vi "DeMux4x4.vi"(1 "Data":bool[](array[boolean]), 2 "Select":bool[](array[boolean])) -> (0 "A":bool[][](array[boolean]))   [LabVIEW 2012]
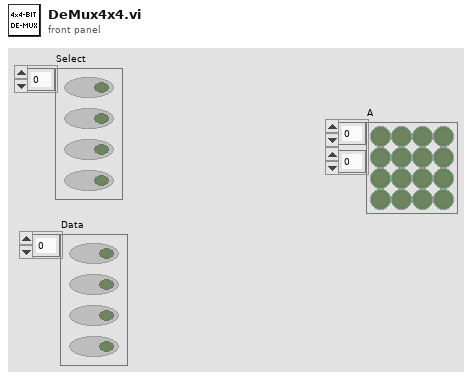
[diagram p1: front panel]
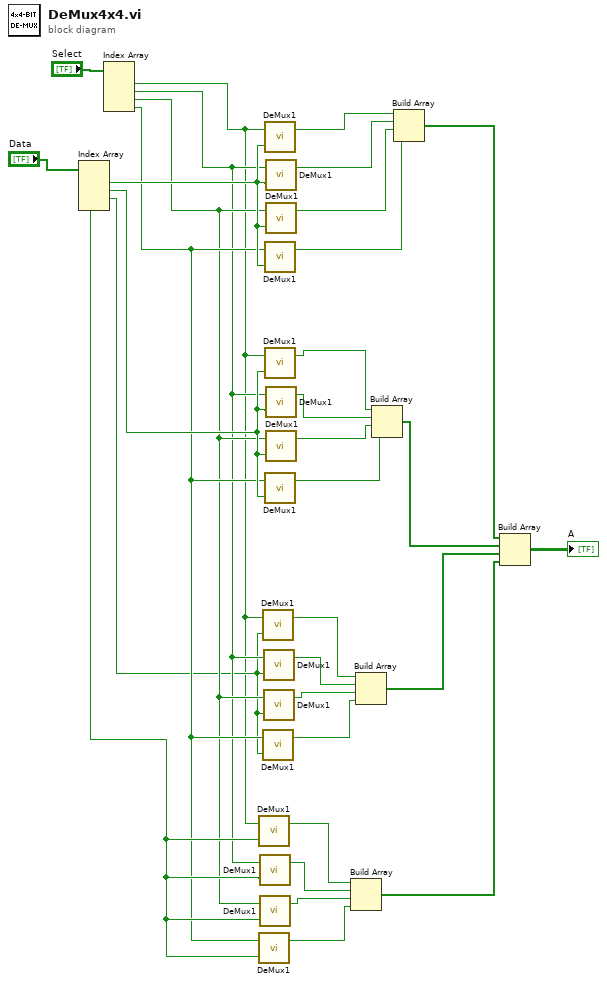
[diagram p0: block diagram]
diagram:
  n1 = Index Array(array="Data") -> (element #1=w25:bool, element #2=w24:bool, element #3=w19:bool, element #4=w23:bool)  [unwired: 4 in]
  n2 = Index Array(array="Select") -> (element #1=w18:bool, element #2=w20:bool, element #3=w21:bool, element #4=w22:bool)  [unwired: 4 in]
  n3 = call "DeMux1.vi"("X"=w23, "S"=w18) -> ("A"=w9:bool)  [unwired: 1 out]
  n4 = call "DeMux1.vi"("X"=w23, "S"=w22) -> ("A"=w6:bool)  [unwired: 1 out]
  n5 = call "DeMux1.vi"("X"=w23, "S"=w20) -> ("A"=w8:bool)  [unwired: 1 out]
  n6 = call "DeMux1.vi"("X"=w23, "S"=w21) -> ("A"=w7:bool)  [unwired: 1 out]
  n7 = call "DeMux1.vi"("X"=w19, "S"=w18) -> ("A"=w13:bool)  [unwired: 1 out]
  n8 = call "DeMux1.vi"("X"=w19, "S"=w22) -> ("A"=w10:bool)  [unwired: 1 out]
  n9 = call "DeMux1.vi"("X"=w19, "S"=w20) -> ("A"=w12:bool)  [unwired: 1 out]
  n10 = call "DeMux1.vi"("X"=w19, "S"=w21) -> ("A"=w11:bool)  [unwired: 1 out]
  n11 = call "DeMux1.vi"("X"=w25, "S"=w18) -> ("A"=w30:bool)  [unwired: 1 out]
  n12 = call "DeMux1.vi"("X"=w25, "S"=w22) -> ("A"=w27:bool)  [unwired: 1 out]
  n13 = call "DeMux1.vi"("X"=w24, "S"=w18) -> ("A"=w17:bool)  [unwired: 1 out]
  n14 = call "DeMux1.vi"("X"=w24, "S"=w22) -> ("A"=w14:bool)  [unwired: 1 out]
  n15 = call "DeMux1.vi"("X"=w25, "S"=w20) -> ("A"=w29:bool)  [unwired: 1 out]
  n16 = call "DeMux1.vi"("X"=w25, "S"=w21) -> ("A"=w28:bool)  [unwired: 1 out]
  n17 = call "DeMux1.vi"("X"=w24, "S"=w20) -> ("A"=w16:bool)  [unwired: 1 out]
  n18 = call "DeMux1.vi"("X"=w24, "S"=w21) -> ("A"=w15:bool)  [unwired: 1 out]
  n19 = Build Array(w9, w8, w7, w6) -> (w2:bool[])
  n20 = Build Array(w13, w12, w11, w10) -> (w3:bool[])
  n21 = Build Array(w17, w16, w15, w14) -> (w4:bool[])
  n22 = Build Array(w30, w29, w28, w27) -> (w5:bool[])
  n23 = Build Array(w5, w4, w3, w2) -> (→"A":bool[][])
